vi "cw_5_2b.vi"() -> ()   [LabVIEW 2022 SP3]
uses:
  <vilib>/Utility/file.llb/Read Delimited Spreadsheet (string).vi
panel:
  out "String":string
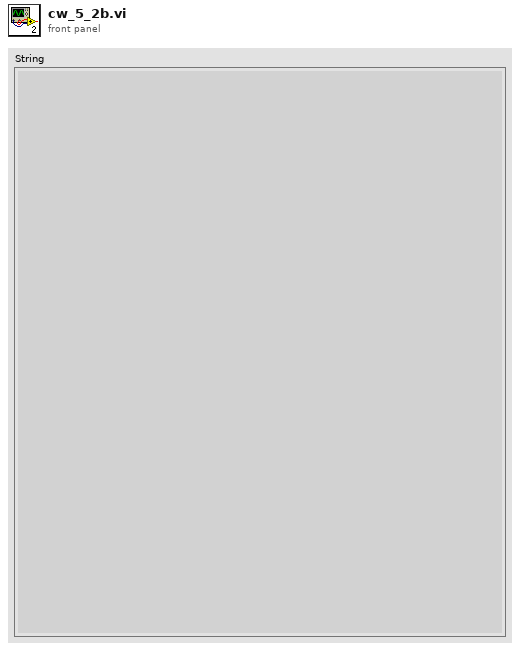
[diagram p1: front panel]
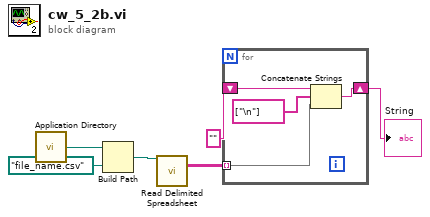
[diagram p0: block diagram]
diagram:
  n1 = call <vilib>:"Application Directory.vi"() -> ("Application Directory"=w6:path)
  n2 = Build Path(base path=w6, name or relative path=path "file_name.csv") -> (appended path=w4:path)
  n3 = call-poly <vilib>:"Read Delimited Spreadsheet.vi"("file path (dialog if empty)"=w4) -> ("all rows"=w3:string[][])  [unwired: 9 in, 5 out]
  n4 = for {
    tunnel: w3 -> [w7] mode=indexing
    shift-right: [w9] -> w1
    shift-left: "" -> [w10]
    n5 = Concatenate Strings(w10, string[] ["\n"] ("string"), w7) -> (w9:string)
  }
  "String" <- w1
